vi "PlainTextToVariant.vi"(7 "use system decimal point (T)":bool=TRUE, 11 "String-formatted Value":string) -> (2 "Value Class":T1, 3 "Variant-formatted Value":variant)   [LabVIEW 2013, in "OpenSerializer.lvlib" / "Serializer.PlainText.lvclass"]
uses:
  Serializer.PlainText.lvclass
  Character Class -- Enum.ctl
  <vilib>/LabVIEW Open Source Project/Data Manipulation/Variant/Variant_EmptyCluster.vi
  <vilib>/Utility/GetType.llb/TD_Create Cluster.vi
  <vilib>/LabVIEW Open Source Project/Data Manipulation/Variant/OpenVariant.lvlib
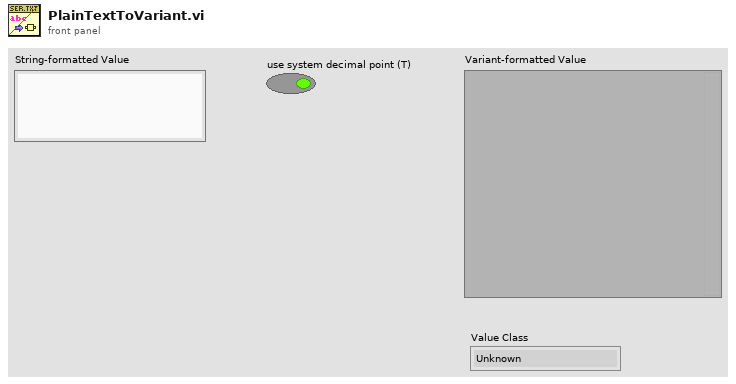
[diagram p1: front panel]
types:
  T1 = typedef "OpenSerializer.lvlib/Serializer.PlainText.lvclass/Character Class -- Enum.ctl" = enum16{"Unknown", "Sign", "Zero", "Integer", "Float", "Complex", "Scientific", "Engineering", "Hexadecimal", "Binary", "Decimal", "Octal", "Unit", "Invalid", "Timestamp", "Boolean", "String", "Path", "null", "cluster", "array"}
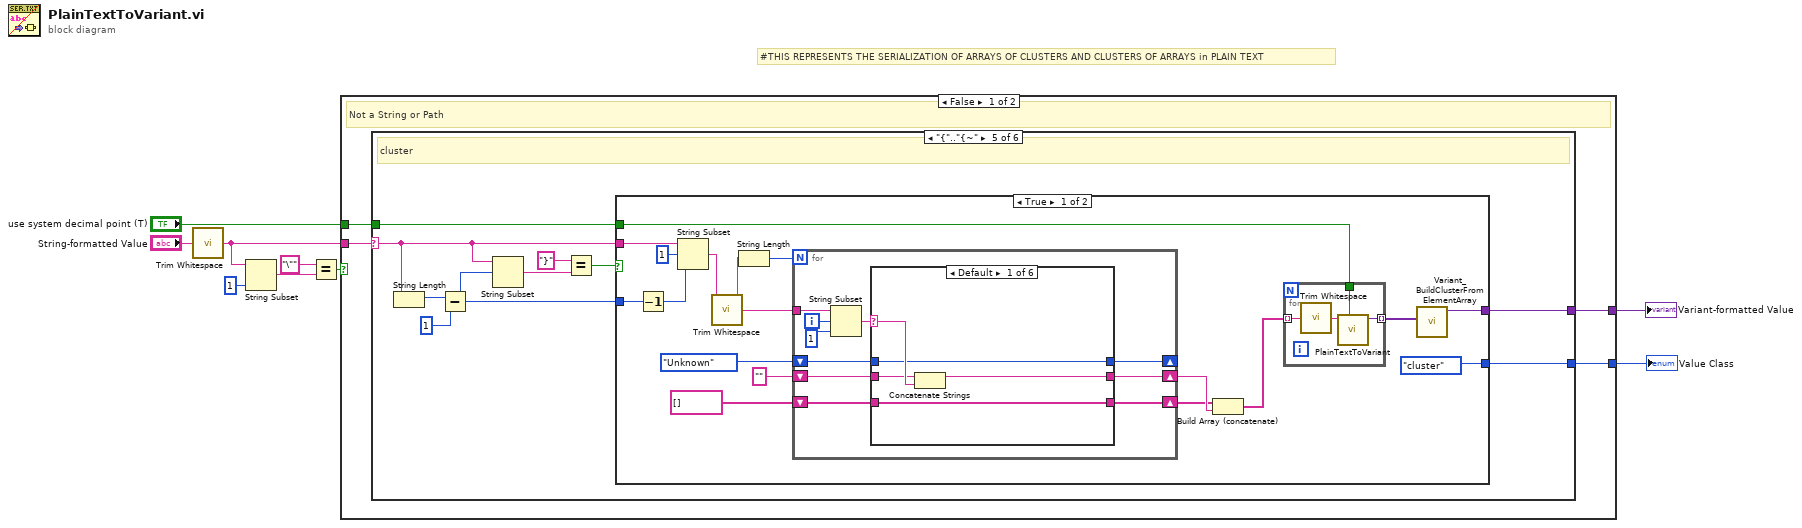
[diagram p0: block diagram]
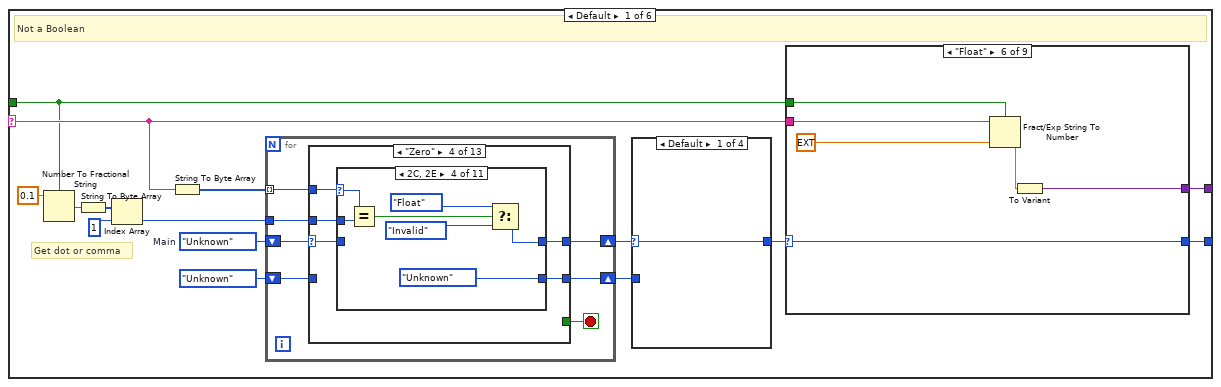
[diagram p2: hidden frame]
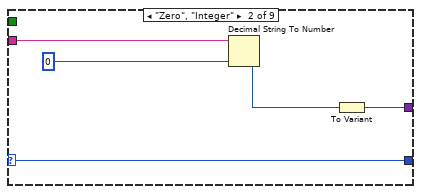
[diagram p4: hidden frame]
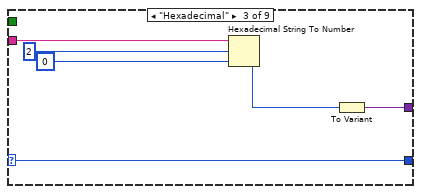
[diagram p5: hidden frame]
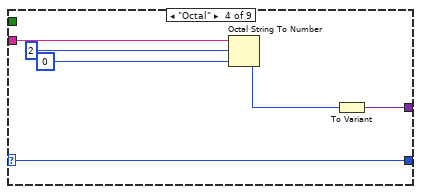
[diagram p6: hidden frame]
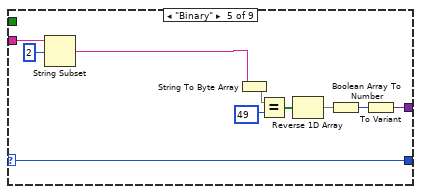
[diagram p7: hidden frame]
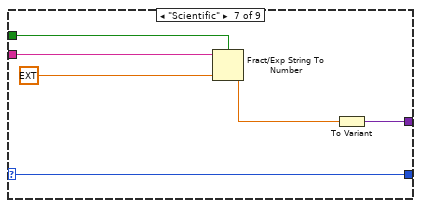
[diagram p8: hidden frame]
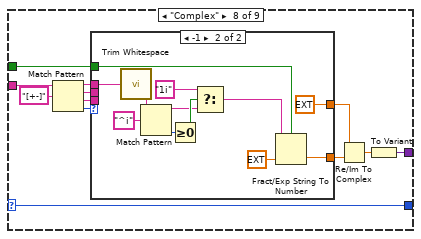
[diagram p9: hidden frame]
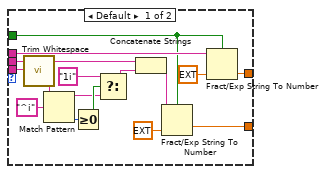
[diagram p10: hidden frame]
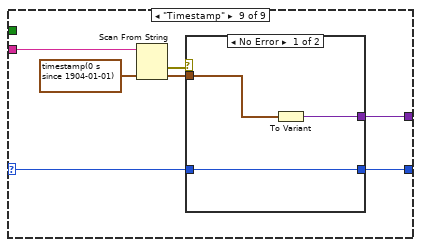
[diagram p11: hidden frame]
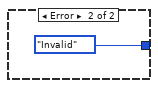
[diagram p12: hidden frame]
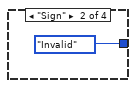
[diagram p13: hidden frame]
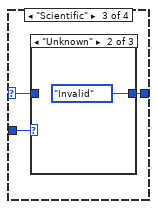
[diagram p14: hidden frame]
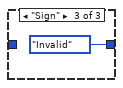
[diagram p16: hidden frame]
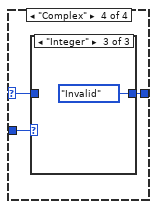
[diagram p17: hidden frame]
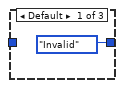
[diagram p18: hidden frame]
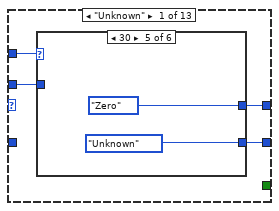
[diagram p20: hidden frame]
diagram:
  # "#THIS REPRESENTS THE SERIALIZATION OF ARRAYS OF CLUSTERS AND CLUSTERS OF ARRAYS in PLAIN TEXT"
  n1 = call <vilib>:"Trim Whitespace.vi"("string"="String-formatted Value") -> ("trimmed string"=w8:string)  [unwired: 1 in]
  n2 = String Subset(string=w8, length (rest)=1 ("length (rest)")) -> (substring=w6:string)  [unwired: 1 in]
  n3 = Equal?(x="\"", y=w6) -> (x = y?=w4:bool)
  n4 = case shown="False" w4 {
    tunnel: w8 -> [w13 w620]
    tunnel: [w12 w628] -> w9
    tunnel: [w11 w621] -> w3
    tunnel: "use system decimal point (T)" -> [w10 _]
    frame False {
      # "Not a String or Path"
      n5 = case shown="\"{\"..\"{~\"" w13 {
        selector: w13 -> [w23 _ _ _ w387 w507]
        tunnel: [w22 w374 w377 w381 w391 w511] -> w12
        tunnel: [w21 Character_Class_--_Enum."Boolean" Character_Class_--_Enum."Boolean" Character_Class_--_Enum."null" w390 w510] -> w11
        tunnel: w10 -> [w18 _ _ _ w382 w502]
        frame Default {
          w27 = Character_Class_--_Enum."Unknown"  # Main
          # "Get dot or comma"
          # "Not a Boolean"
          n6 = Number To Fractional String(use system decimal point (T)=w18, number=0.1) -> (F-format string=w16:string)  [unwired: 2 in]
          n7 = String To Byte Array(string=w16) -> (unsigned byte array=w17:u8[])
          n8 = Index Array(array=w17, index=1 ("length (rest)")) -> (element=w14:u8)
          n9 = String To Byte Array(string=w23) -> (unsigned byte array=w28:u8[])
          n10 = for {
            tunnel: w28 -> [w139] mode=indexing
            shift-right: [w138] -> w26
            shift-left: w27 -> [w140]
            shift-right: [w136] -> w25
            shift-left: Character_Class_--_Enum."Unknown" -> [w137]
            tunnel: w14 -> [w134]
            stop <- w135 stop-if-true
            n11 = case shown="\"Zero\"" w140 {
              selector: w140 -> [_ w163 w167 w186 w217 w240 w246 w252 w258 w264 w267 w283 w324]
              tunnel: w139 -> [w144 _ w169 w188 w219 w242 w248 w254 w260 _ w269 w285 w326]
              tunnel: [w143 w163 w168 w187 w218 w241 w247 w253 w259 w264 w268 w284 w325] -> w138
              tunnel: w137 -> [_ w162 w164 _ _ _ _ _ _ _ _ w282 w323]
              tunnel: [w142 w162 w165 w185 w216 Character_Class_--_Enum."Unknown" Character_Class_--_Enum."Unknown" Character_Class_--_Enum."Unknown" Character_Class_--_Enum."Unknown" Character_Class_--_Enum."Unknown" w266 w281 w322] -> w136
              tunnel: [_ TRUE _ _ _ _ _ _ _ TRUE _ _ _] -> w135
              tunnel: w134 -> [w141 _ w166 w184 w215 _ _ _ _ _ _ _ w321]
              frame "Unknown" {
                n12 = case shown="30" w144 {
                  selector: w144 -> [_ _ _ w155 _ _]
                  tunnel: [Character_Class_--_Enum."Invalid" Character_Class_--_Enum."Sign" Character_Class_--_Enum."Integer" w151 Character_Class_--_Enum."Zero" w160] -> w143
                  tunnel: [Character_Class_--_Enum."Unknown" Character_Class_--_Enum."Unknown" Character_Class_--_Enum."Unknown" Character_Class_--_Enum."Unknown" Character_Class_--_Enum."Unknown" w160] -> w142
                  tunnel: w141 -> [_ _ _ w156 _ _]
                  frame Default {
                  }
                  frame 43, 45 {
                  }
                  frame 49..57 {
                  }
                  frame 44, 46 {
                    n13 = Equal?(x=w155, y=w156) -> (x = y?=w154:bool)
                    n14 = Select(t=Character_Class_--_Enum."Float", s=w154, f=Character_Class_--_Enum."Invalid") -> (s? t:f=w151:T1)
                  }
                  frame 48 {
                  }
                  frame 105 {
                    w160 = Character_Class_--_Enum."Complex"
                  }
                }
              }
              frame "Invalid", Default {
              }
              frame "Sign" {
                n15 = case shown="69" w169 {
                  selector: w169 -> [_ _ _ _ w180]
                  tunnel: [Character_Class_--_Enum."Invalid" w173 Character_Class_--_Enum."Integer" w176 w178] -> w168
                  tunnel: w167 -> [_ w173 _ _ _]
                  tunnel: w166 -> [_ _ _ _ w179]
                  tunnel: [Character_Class_--_Enum."Unknown" w172 Character_Class_--_Enum."Unknown" w176 Character_Class_--_Enum."Unknown"] -> w165
                  tunnel: w164 -> [_ w172 _ _ _]
                  frame Default {
                  }
                  frame 32 {
                    # "space (ignore)"
                  }
                  frame 48..57 {
                  }
                  frame 105 {
                    w176 = Character_Class_--_Enum."Complex"
                  }
                  frame 44, 46 {
                    n16 = Equal?(x=w180, y=w179) -> (x = y?=w183:bool)
                    n17 = Select(t=Character_Class_--_Enum."Float", s=w183, f=Character_Class_--_Enum."Invalid") -> (s? t:f=w178:T1)
                  }
                }
              }
              frame "Zero" {
                n18 = case shown="2C, 2E" w188 {
                  selector: w188 -> [_ _ _ w196 _ _ _ _ _ _ _]
                  tunnel: [Character_Class_--_Enum."Invalid" Character_Class_--_Enum."Integer" w194 w195 Character_Class_--_Enum."Hexadecimal" Character_Class_--_Enum."Binary" Character_Class_--_Enum."Octal" Character_Class_--_Enum."Decimal" w211 w212 Character_Class_--_Enum."Complex"] -> w187
                  tunnel: w186 -> [_ _ w194 _ _ _ _ _ w211 _ _]
                  tunnel: [Character_Class_--_Enum."Unknown" Character_Class_--_Enum."Unknown" Character_Class_--_Enum."Unknown" Character_Class_--_Enum."Unknown" Character_Class_--_Enum."Unknown" Character_Class_--_Enum."Unknown" Character_Class_--_Enum."Unknown" Character_Class_--_Enum."Unknown" Character_Class_--_Enum."Unknown" w212 Character_Class_--_Enum."Unknown"] -> w185
                  tunnel: w184 -> [_ _ _ w197 _ _ _ _ _ _ _]
                  frame Default {
                  }
                  frame 49..57 {
                  }
                  frame 48 {
                  }
                  frame 44, 46 {
                    n19 = Equal?(x=w196, y=w197) -> (x = y?=w200:bool)
                    n20 = Select(t=Character_Class_--_Enum."Float", s=w200, f=Character_Class_--_Enum."Invalid") -> (s? t:f=w195:T1)
                  }
                  frame 120 {
                  }
                  frame 98 {
                  }
                  frame 111 {
                  }
                  frame 100 {
                  }
                  frame 32 {
                  }
                  frame 105 {
                    w212 = Character_Class_--_Enum."Complex"
                  }
                  frame 43, 45 {
                  }
                }
              }
              frame "Integer" {
                n21 = case shown="3A" w219 {
                  selector: w219 -> [_ _ _ _ _ w230 _ _]
                  tunnel: [Character_Class_--_Enum."Invalid" w222 w223 w225 w227 w228 Character_Class_--_Enum."Complex" Character_Class_--_Enum."Scientific"] -> w218
                  tunnel: w217 -> [_ _ _ w225 w227 _ _ _]
                  tunnel: [Character_Class_--_Enum."Unknown" w222 w223 Character_Class_--_Enum."Unknown" Character_Class_--_Enum."Unknown" Character_Class_--_Enum."Unknown" Character_Class_--_Enum."Unknown" Character_Class_--_Enum."Unknown"] -> w216
                  tunnel: w215 -> [_ _ _ _ _ w229 _ _]
                  frame Default {
                  }
                  frame 105 {
                    w222 = Character_Class_--_Enum."Complex"
                  }
                  frame 58 {
                    w223 = Character_Class_--_Enum."Timestamp"
                  }
                  frame 32 {
                  }
                  frame 48..57 {
                  }
                  frame 44, 46 {
                    n22 = Equal?(x=w230, y=w229) -> (x = y?=w233:bool)
                    n23 = Select(t=Character_Class_--_Enum."Float", s=w233, f=Character_Class_--_Enum."Invalid") -> (s? t:f=w228:T1)
                  }
                  frame 43, 45 {
                  }
                  frame 69, 101 {
                  }
                }
              }
              frame "Hexadecimal" {
                n24 = case shown="30..39, 41..46" w242 {
                  tunnel: [Character_Class_--_Enum."Invalid" w244] -> w241
                  tunnel: w240 -> [_ w244]
                  frame Default {
                  }
                  frame 48..57, 65..70 {
                  }
                }
              }
              frame "Decimal" {
                n25 = case shown="30..39" w248 {
                  tunnel: [Character_Class_--_Enum."Invalid" w250] -> w247
                  tunnel: w246 -> [_ w250]
                  frame Default {
                  }
                  frame 48..57 {
                  }
                }
              }
              frame "Octal" {
                n26 = case shown="30..37" w254 {
                  tunnel: [Character_Class_--_Enum."Invalid" w256] -> w253
                  tunnel: w252 -> [_ w256]
                  frame Default {
                  }
                  frame 48..55 {
                  }
                }
              }
              frame "Binary" {
                n27 = case shown="30, 31" w260 {
                  tunnel: [Character_Class_--_Enum."Invalid" w262] -> w259
                  tunnel: w258 -> [_ w262]
                  frame Default {
                  }
                  frame 48, 49 {
                  }
                }
              }
              frame "Timestamp" {
              }
              frame "Float" {
                n28 = case shown="2B, 2D" w269 {
                  tunnel: [Character_Class_--_Enum."Invalid" w273 Character_Class_--_Enum."Scientific" w277 Character_Class_--_Enum."Complex" w280] -> w268
                  tunnel: w267 -> [_ w273 _ w277 _ _]
                  tunnel: [Character_Class_--_Enum."Unknown" Character_Class_--_Enum."Unknown" Character_Class_--_Enum."Unknown" Character_Class_--_Enum."Unknown" Character_Class_--_Enum."Unknown" w280] -> w266
                  frame Default {
                  }
                  frame 48..57 {
                  }
                  frame 69, 101 {
                  }
                  frame 32 {
                  }
                  frame 43, 45 {
                  }
                  frame 105 {
                    w280 = Character_Class_--_Enum."Complex"
                  }
                }
              }
              frame "Scientific" {
                n29 = case shown="2B, 2D" w285 {
                  tunnel: [Character_Class_--_Enum."Invalid" w289 w301 w314] -> w284
                  tunnel: w283 -> [_ w288 w303 w316]
                  tunnel: w282 -> [w286 w290 w302 w315]
                  tunnel: [w286 w291 w304 w317] -> w281
                  frame Default {
                  }
                  frame 49..57 {
                    n30 = case shown="\"Unknown\"" w290 {
                      selector: w290 -> [_ _ _ w297 _]
                      tunnel: [w292 Character_Class_--_Enum."Integer" Character_Class_--_Enum."Integer" w297 Character_Class_--_Enum."Integer"] -> w291
                      tunnel: [w292 w293 w296 w298 w300] -> w289
                      tunnel: w288 -> [_ w293 w296 w298 w300]
                      frame Default {
                        w292 = Character_Class_--_Enum."Invalid"
                      }
                      frame "Sign" {
                      }
                      frame "Zero" {
                      }
                      frame "Integer" {
                      }
                      frame "Unknown" {
                      }
                    }
                  }
                  frame 48 {
                    n31 = case shown="\"Sign\"" w302 {
                      tunnel: [w305 Character_Class_--_Enum."Zero" Character_Class_--_Enum."Zero" Character_Class_--_Enum."Zero" Character_Class_--_Enum."Integer"] -> w304
                      tunnel: w303 -> [_ w306 w308 w310 w312]
                      tunnel: [w305 w306 w308 w310 w312] -> w301
                      frame Default {
                        w305 = Character_Class_--_Enum."Invalid"
                      }
                      frame "Unknown" {
                      }
                      frame "Sign" {
                      }
                      frame "Zero" {
                      }
                      frame "Integer" {
                      }
                    }
                  }
                  frame 43, 45 {
                    n32 = case shown="\"Unknown\"" w315 {
                      tunnel: [w318 Character_Class_--_Enum."Sign"] -> w317
                      tunnel: w316 -> [_ w319]
                      tunnel: [w318 w319] -> w314
                      frame Default {
                        w318 = Character_Class_--_Enum."Invalid"
                      }
                      frame "Unknown" {
                      }
                    }
                  }
                }
              }
              frame "Complex" {
                n33 = case shown="2C, 2E" w326 {
                  selector: w326 -> [_ _ _ w342 _]
                  tunnel: [w327 w329 w332 w345 w364] -> w325
                  tunnel: w324 -> [_ w329 w330 w343 w362]
                  tunnel: w323 -> [_ w328 w333 w346 w365]
                  tunnel: [w327 w328 w331 w344 w363] -> w322
                  tunnel: w321 -> [_ _ _ w341 _]
                  frame Default {
                    w327 = Character_Class_--_Enum."Invalid"
                  }
                  frame 32 {
                  }
                  frame 48..57 {
                    n34 = case shown="Default" w333 {
                      selector: w333 -> [_ _ w337 w339]
                      tunnel: [w334 w336 w338 w340] -> w332
                      tunnel: [w334 Character_Class_--_Enum."Integer" w337 w339] -> w331
                      tunnel: w330 -> [_ w336 w338 w340]
                      frame Default {
                        w334 = Character_Class_--_Enum."Invalid"
                      }
                      frame "Unknown" {
                      }
                      frame "Integer" {
                      }
                      frame "Float" {
                      }
                    }
                  }
                  frame 44, 46 {
                    n35 = case shown="\"Unknown\"" w346 {
                      tunnel: [w347 w354 w361] -> w345
                      tunnel: [w347 w348 w357] -> w344
                      tunnel: w343 -> [_ w354 w361]
                      tunnel: w342 -> [_ w350 w356]
                      tunnel: w341 -> [_ w349 w355]
                      frame Default {
                        w347 = Character_Class_--_Enum."Invalid"
                      }
                      frame "Unknown" {
                        n36 = Equal?(x=w350, y=w349) -> (x = y?=w353:bool)
                        n37 = Select(t=Character_Class_--_Enum."Float", s=w353, f=Character_Class_--_Enum."Invalid") -> (s? t:f=w348:T1)
                      }
                      frame "Integer" {
                        n38 = Equal?(x=w356, y=w355) -> (x = y?=w360:bool)
                        n39 = Select(t=Character_Class_--_Enum."Float", s=w360, f=Character_Class_--_Enum."Invalid") -> (s? t:f=w357:T1)
                      }
                    }
                  }
                  frame 105 {
                    n40 = case shown="\"Float\"" w365 {
                      tunnel: [w366 w368 w370 w372] -> w364
                      tunnel: [w366 Character_Class_--_Enum."Complex" Character_Class_--_Enum."Complex" Character_Class_--_Enum."Complex"] -> w363
                      tunnel: w362 -> [_ w368 w370 w372]
                      frame Default {
                        w366 = Character_Class_--_Enum."Invalid"
                      }
                      frame "Unknown" {
                      }
                      frame "Integer" {
                      }
                      frame "Float" {
                      }
                    }
                  }
                }
              }
            }
          }
          n41 = case shown="Default" w26 {
            selector: w26 -> [w120 _ w122 w128]
            tunnel: w25 -> [_ _ w124 w130]
            tunnel: [w120 Character_Class_--_Enum."Invalid" w123 w129] -> w24
            frame Default {
            }
            frame "Sign" {
            }
            frame "Scientific" {
              n42 = case shown="\"Unknown\"" w124 {
                tunnel: [w125 Character_Class_--_Enum."Invalid" Character_Class_--_Enum."Invalid"] -> w123
                tunnel: w122 -> [w125 _ _]
                frame Default {
                }
                frame "Unknown" {
                }
                frame "Sign" {
                }
              }
            }
            frame "Complex" {
              n43 = case shown="\"Integer\"" w130 {
                tunnel: [Character_Class_--_Enum."Invalid" w132 Character_Class_--_Enum."Invalid" ("Main")] -> w129
                tunnel: w128 -> [_ w132 _]
                frame Default {
                }
                frame "Complex" {
                }
                frame "Integer" {
                }
              }
            }
          }
          n44 = case shown="\"Float\"" w24 {
            selector: w24 -> [w29 w30 w35 w41 w47 w58 w64 w79 w109]
            tunnel: w23 -> [_ w34 w40 w46 w55 w62 w68 w75 w115]
            tunnel: [_ w31 w37 w43 w56 w59 w65 w80 w112] -> w22
            tunnel: [w29 w30 w35 w41 w47 w58 w64 w79 w110] -> w21
            tunnel: w18 -> [_ _ _ _ _ w57 w63 w70 _]
            frame Default {
            }
            frame "Zero", "Integer" {
              n45 = Decimal String To Number(string=w34, default (0L)=i64 0 ("default (0 I32)")) -> (number=w32:i64)  [unwired: 1 in, 1 out]
              n46 = To Variant(anything=w32) -> (Variant=w31:variant)
            }
            frame "Hexadecimal" {
              n47 = Hexadecimal String To Number(string=w40, offset=2, default (0uL)=i64 0 ("default (0 I32)")) -> (number=w38:i64)  [unwired: 1 out]
              n48 = To Variant(anything=w38) -> (Variant=w37:variant)
            }
            frame "Octal" {
              n49 = Octal String To Number(2:i64 0 ("default (0 I32)"), 3:2 ("offset"), 4:w46) -> (0:w44:i64)  [unwired: 1 out]
              n50 = To Variant(anything=w44) -> (Variant=w43:variant)
            }
            frame "Binary" {
              n51 = String Subset(string=w55, offset (0)=2) -> (substring=w53:string)  [unwired: 1 in]
              n52 = String To Byte Array(string=w53) -> (unsigned byte array=w51:u8[])
              n53 = Equal?(x=w51, y=u8 49 ("offset (0)")) -> (x = y?=w50:bool[])
              n54 = Reverse 1D Array(array=w50) -> (reversed array=w48:bool[])
              n55 = Boolean Array To Number(Boolean array=w48) -> (number=w52:u32)
              n56 = To Variant(anything=w52) -> (Variant=w56:variant)
            }
            frame "Float" {
              n57 = Fract/Exp String To Number(use system decimal point (T)=w57, string=w62, default (0 dbl)=ext 0.0 ("default (0 I32)")) -> (number=w60:ext)  [unwired: 1 in, 1 out]
              n58 = To Variant(anything=w60) -> (Variant=w59:variant)
            }
            frame "Scientific" {
              n59 = Fract/Exp String To Number(use system decimal point (T)=w63, string=w68, default (0 dbl)=ext 0.0 ("default (0 I32)")) -> (number=w66:ext)  [unwired: 1 in, 1 out]
              n60 = To Variant(anything=w66) -> (Variant=w65:variant)
            }
            frame "Complex" {
              n61 = Match Pattern(string=w75, regular expression="[+-]") -> (before substring=w72:string, match substring=w69:string, after substring=w71:string, offset past match=w76:i32)  [unwired: 1 in]
              n62 = case shown="-1" w76 {
                tunnel: [w93 ext 0.0 ("default (0 DBL)")] -> w73
                tunnel: [w95 w106] -> w74
                tunnel: w72 -> [w92 w98]
                tunnel: w71 -> [w82 _]
                tunnel: w70 -> [w91 w105]
                tunnel: w69 -> [w85 _]
                frame Default {
                  n63 = call <vilib>:"Trim Whitespace.vi"("string"=w82) -> ("trimmed string"=w83:string)  [unwired: 1 in]
                  n64 = Match Pattern(string=w83, regular expression="^i") -> (before substring=w88:string, offset past match=w90:i32)  [unwired: 1 in, 2 out]
                  n65 = Greater Or Equal To 0?(x=w90) -> (x >= 0?=w89:bool)
                  n66 = Select(t="1i", s=w89, f=w88) -> (s? t:f=w86:string)
                  n67 = Concatenate Strings(w85, w86) -> (w84:string)
                  n68 = Fract/Exp String To Number(use system decimal point (T)=w91, string=w84, default (0 dbl)=ext 0.0 ("default (0 DBL)")) -> (number=w95:ext)  [unwired: 1 in, 1 out]
                  n69 = Fract/Exp String To Number(use system decimal point (T)=w91, string=w92, default (0 dbl)=ext 0.0 ("default (0 DBL)")) -> (number=w93:ext)  [unwired: 1 in, 1 out]
                }
                frame -1 {
                  n70 = call <vilib>:"Trim Whitespace.vi"("string"=w98) -> ("trimmed string"=w100:string)  [unwired: 1 in]
                  n71 = Match Pattern(string=w100, regular expression="^i") -> (before substring=w102:string, offset past match=w104:i32)  [unwired: 1 in, 2 out]
                  n72 = Greater Or Equal To 0?(x=w104) -> (x >= 0?=w103:bool)
                  n73 = Select(t="1i", s=w103, f=w102) -> (s? t:f=w97:string)
                  n74 = Fract/Exp String To Number(use system decimal point (T)=w105, string=w97, default (0 dbl)=ext 0.0 ("default (0 DBL)")) -> (number=w106:ext)  [unwired: 1 in, 1 out]
                }
              }
              n75 = Re/Im To Complex(1:w74, 2:w73) -> (0:w78:cxt)
              n76 = To Variant(anything=w78) -> (Variant=w80:variant)
            }
            frame "Timestamp" {
              n77 = Scan From String(input string=w115, default 1=timestamp(0 s since 1904-01-01)) -> (error out=w111:errorcluster, output 1=w113:timestamp)  [unwired: 3 in, 2 out]
              n78 = case shown="No Error" w111 {
                tunnel: w113 -> [w118 _]
                tunnel: [w117 _] -> w112
                tunnel: [w116 Character_Class_--_Enum."Invalid"] -> w110
                tunnel: w109 -> [w116 _]
                frame No Error {
                  n79 = To Variant(anything=w118) -> (Variant=w117:variant)
                }
                frame Error {
                }
              }
            }
          }
        }
        frame "true" {
          # "BOOLEAN (TRUE)"
          n80 = To Variant(anything=TRUE) -> (Variant=w374:variant)
        }
        frame "false" {
          # "BOOLEAN (FALSE)"
          n81 = To Variant(anything=FALSE) -> (Variant=w377:variant)
        }
        frame "null" {
          # "null"
          n82 = To Variant(anything=variant ("variant")) -> (Variant=w381:variant)
        }
        frame "{".."{~" {
          # "cluster"
          n83 = String Length(string=w387) -> (length=w389:i32)
          n84 = Subtract(x=w389, y=1) -> (x-y=w383:i32)
          n85 = String Subset(string=w387, offset (0)=w383) -> (substring=w385:string)  [unwired: 1 in]
          n86 = Equal?(x="}", y=w385) -> (x = y?=w384:bool)
          n87 = case shown="True" w384 {
            tunnel: [w400 w501] -> w391
            tunnel: [Character_Class_--_Enum."cluster" Character_Class_--_Enum."Invalid"] -> w390
            tunnel: w387 -> [w407 _]
            tunnel: w383 -> [w405 _]
            tunnel: w382 -> [w402 _]
            frame True {
              n88 = Decrement(x=w405) -> (x-1=w404:i32)
              n89 = String Subset(string=w407, offset (0)=1, length (rest)=w404) -> (substring=w403:string)
              n90 = call <vilib>:"Trim Whitespace.vi"("string"=w403) -> ("trimmed string"=w397:string)  [unwired: 1 in]
              n91 = String Length(string=w397) -> (length=w398:i32)
              n92 = for {
                N: w398 -> [_]
                shift-right: [w412] -> w394
                shift-left: string[] [] -> [w413]
                tunnel: w397 -> [w418]
                shift-right: [w411] -> w395
                shift-left: "" -> [w414]
                shift-right: [w409] -> _
                shift-left: Character_Class_--_Enum."Unknown" -> [w410]
                i -> [w417]
                n93 = String Subset(string=w418, offset (0)=w417, length (rest)=1 ("offset (0)")) -> (substring=w415:string)
                n94 = case shown="Default" w415 {
                  selector: w415 -> [w422 w425 w443 w455 w469 w483]
                  tunnel: w414 -> [w421 w430 w444 w456 w470 w484]
                  tunnel: w413 -> [w423 w429 w446 w458 w472 w486]
                  tunnel: [w423 w428 w446 w458 w472 w486] -> w412
                  tunnel: [w420 w427 w442 w454 w468 w482] -> w411
                  tunnel: w410 -> [w419 w426 w445 w457 w471 w485]
                  tunnel: [w419 w424 w441 w453 w467 w481] -> w409
                  frame Default {
                    n95 = Concatenate Strings(w421, w422) -> (w420:string)
                  }
                  frame "," {
                    n96 = case shown="\"Unknown\", Default" w426 {
                      selector: w426 -> [w431 w436]
                      tunnel: w430 -> [w435 w439]
                      tunnel: w429 -> [w434 w440]
                      tunnel: [w433 w440] -> w428
                      tunnel: ["" w437] -> w427
                      tunnel: w425 -> [_ w438]
                      tunnel: [w431 w436] -> w424
                      frame "Unknown", Default {
                        n97 = Build Array (concatenate)(w434, w435) -> (w433:string[])
                      }
                      frame "cluster", "array" {
                        n98 = Concatenate Strings(w439, w438) -> (w437:string)
                      }
                    }
                  }
                  frame "{" {
                    n99 = case shown="Default" w445 {
                      selector: w445 -> [_ w449]
                      tunnel: w444 -> [_ w452]
                      tunnel: w443 -> [w447 w451]
                      tunnel: [w447 w450] -> w442
                      tunnel: [Character_Class_--_Enum."cluster" w449] -> w441
                      frame Default {
                      }
                      frame "cluster" {
                        n100 = Concatenate Strings(w452, w451) -> (w450:string)
                      }
                    }
                  }
                  frame "}" {
                    n101 = case shown="\"cluster\"" w457 {
                      selector: w457 -> [w459 _]
                      tunnel: w456 -> [w462 w464]
                      tunnel: w455 -> [w461 w465]
                      tunnel: [w460 w463] -> w454
                      tunnel: [w459 Character_Class_--_Enum."Unknown"] -> w453
                      frame Default {
                        n102 = Concatenate Strings(w462, w461) -> (w460:string)
                      }
                      frame "cluster" {
                        n103 = Concatenate Strings(w464, w465) -> (w463:string)
                      }
                    }
                  }
                  frame "[" {
                    n104 = case shown="Default" w471 {
                      tunnel: w470 -> [w476 w478]
                      tunnel: w469 -> [w475 w479]
                      tunnel: [w474 w477] -> w468
                      tunnel: [Character_Class_--_Enum."array" Character_Class_--_Enum."array"] -> w467
                      frame Default {
                        n105 = Concatenate Strings(w476, w475) -> (w474:string)
                      }
                      frame "cluster" {
                        n106 = Concatenate Strings(w478, w479) -> (w477:string)
                      }
                    }
                  }
                  frame "]" {
                    n107 = case shown="\"array\"" w485 {
                      selector: w485 -> [w487 _]
                      tunnel: w484 -> [w490 w492]
                      tunnel: w483 -> [w489 w493]
                      tunnel: [w488 w491] -> w482
                      tunnel: [w487 Character_Class_--_Enum."Unknown"] -> w481
                      frame Default {
                        n108 = Concatenate Strings(w490, w489) -> (w488:string)
                      }
                      frame "array" {
                        n109 = Concatenate Strings(w492, w493) -> (w491:string)
                      }
                    }
                  }
                }
              }
              n110 = Build Array (concatenate)(w394, w395) -> (w393:string[])
              n111 = for {
                tunnel: w402 -> [w498]
                tunnel: w393 -> [w497] mode=indexing
                tunnel: [w495] -> w401 mode=indexing
                n112 = call <vilib>:"Trim Whitespace.vi"("string"=w497) -> ("trimmed string"=w496:string)  [unwired: 1 in]
                n113 = call "PlainTextToVariant.vi"("use system decimal point (T)"=w498, "String-formatted Value"=w496) -> ("Variant-formatted Value"=w495:variant)  [unwired: 8 in, 1 out]
              }
              n114 = call <vilib>:"Variant_BuildClusterFromElementArray.vi"("Elements"=w401) -> ("Cluster"=w400:variant)  [unwired: 10 in]
            }
            frame False {
              n115 = To Variant(anything=variant ("variant")) -> (Variant=w501:variant)
            }
          }
        }
        frame "[".."[~" {
          # "array"
          n116 = String Length(string=w507) -> (length=w509:i32)
          n117 = Subtract(x=w509, y=1) -> (x-y=w503:i32)
          n118 = String Subset(string=w507, offset (0)=w503) -> (substring=w505:string)  [unwired: 1 in]
          n119 = Equal?(x="]", y=w505) -> (x = y?=w504:bool)
          n120 = case shown="True" w504 {
            tunnel: [w515 w619] -> w511
            tunnel: [Character_Class_--_Enum."array" Character_Class_--_Enum."Invalid"] -> w510
            tunnel: w507 -> [w513 _]
            tunnel: w503 -> [w526 _]
            tunnel: w502 -> [w524 _]
            frame True {
              # "#THIS IS UPDATED AS WELL\nto support undefined array input"
              n121 = Decrement(x=w526) -> (x-1=w525:i32)
              n122 = String Subset(string=w513, offset (0)=1, length (rest)=w525) -> (substring=w512:string)
              n123 = call <vilib>:"Trim Whitespace.vi"("string"=w512) -> ("trimmed string"=w521:string)  [unwired: 1 in]
              n124 = String Length(string=w521) -> (length=w522:i32)
              n125 = for {
                N: w522 -> [_]
                shift-right: [w532] -> w518
                shift-left: string[] [] -> [w533]
                tunnel: w521 -> [w538]
                shift-right: [w531] -> w519
                shift-left: "" -> [w534]
                shift-right: [w529] -> _
                shift-left: Character_Class_--_Enum."Unknown" -> [w530]
                i -> [w537]
                n126 = String Subset(string=w538, offset (0)=w537, length (rest)=1 ("offset (0)")) -> (substring=w535:string)
                n127 = case shown="\"]\"" w535 {
                  selector: w535 -> [w542 w545 w563 w575 w587 w601]
                  tunnel: w534 -> [w541 w550 w564 w576 w588 w602]
                  tunnel: w533 -> [w543 w549 w566 w578 w590 w604]
                  tunnel: [w543 w548 w566 w578 w590 w604] -> w532
                  tunnel: [w540 w547 w562 w574 w586 w600] -> w531
                  tunnel: w530 -> [w539 w546 w565 w577 w589 w603]
                  tunnel: [w539 w544 w561 w573 w585 w599] -> w529
                  frame Default {
                    n128 = Concatenate Strings(w541, w542) -> (w540:string)
                  }
                  frame "," {
                    n129 = case shown="\"cluster\"" w546 {
                      selector: w546 -> [w551 w556]
                      tunnel: w550 -> [w555 w559]
                      tunnel: w549 -> [w554 w560]
                      tunnel: [w553 w560] -> w548
                      tunnel: ["" w557] -> w547
                      tunnel: w545 -> [_ w558]
                      tunnel: [w551 w556] -> w544
                      frame "Unknown", Default {
                        n130 = Build Array (concatenate)(w554, w555) -> (w553:string[])
                      }
                      frame "cluster" {
                        n131 = Concatenate Strings(w559, w558) -> (w557:string)
                      }
                    }
                  }
                  frame "[" {
                    n132 = case shown="\"array\"" w565 {
                      selector: w565 -> [_ w569]
                      tunnel: w564 -> [_ w572]
                      tunnel: w563 -> [w567 w571]
                      tunnel: [w567 w570] -> w562
                      tunnel: [Character_Class_--_Enum."array" w569] -> w561
                      frame Default {
                      }
                      frame "array" {
                        n133 = Concatenate Strings(w572, w571) -> (w570:string)
                      }
                    }
                  }
                  frame "{" {
                    n134 = case shown="Default" w577 {
                      selector: w577 -> [_ w581]
                      tunnel: w576 -> [_ w584]
                      tunnel: w575 -> [w579 w583]
                      tunnel: [w579 w582] -> w574
                      tunnel: [Character_Class_--_Enum."cluster" w581] -> w573
                      frame Default {
                      }
                      frame "cluster" {
                        n135 = Concatenate Strings(w584, w583) -> (w582:string)
                      }
                    }
                  }
                  frame "]" {
                    n136 = case shown="\"array\"" w589 {
                      selector: w589 -> [w591 _]
                      tunnel: w588 -> [w594 w596]
                      tunnel: w587 -> [w593 w597]
                      tunnel: [w592 w595] -> w586
                      tunnel: [w591 Character_Class_--_Enum."Unknown"] -> w585
                      frame Default {
                        n137 = Concatenate Strings(w594, w593) -> (w592:string)
                      }
                      frame "array" {
                        n138 = Concatenate Strings(w596, w597) -> (w595:string)
                      }
                    }
                  }
                  frame "}" {
                    n139 = case shown="\"cluster\"" w603 {
                      selector: w603 -> [w605 _]
                      tunnel: w602 -> [w608 w610]
                      tunnel: w601 -> [w607 w611]
                      tunnel: [w606 w609] -> w600
                      tunnel: [w605 Character_Class_--_Enum."Unknown"] -> w599
                      frame Default {
                        n140 = Concatenate Strings(w608, w607) -> (w606:string)
                      }
                      frame "cluster" {
                        n141 = Concatenate Strings(w610, w611) -> (w609:string)
                      }
                    }
                  }
                }
              }
              n142 = Build Array (concatenate)(w518, w519) -> (w517:string[])
              n143 = for {
                tunnel: w524 -> [w616]
                tunnel: w517 -> [w615] mode=indexing
                tunnel: [w613] -> w514 mode=indexing
                n144 = call <vilib>:"Trim Whitespace.vi"("string"=w615) -> ("trimmed string"=w614:string)  [unwired: 1 in]
                n145 = call "PlainTextToVariant.vi"("use system decimal point (T)"=w616, "String-formatted Value"=w614) -> ("Variant-formatted Value"=w613:variant)  [unwired: 8 in, 1 out]
              }
              n146 = call <vilib>:"Variant_BuildArrayFromElementArray.vi"("Elements"=w514) -> ("Output Array"=w515:variant)  [unwired: 9 in, 1 out]
            }
            frame False {
              n147 = To Variant(anything=variant ("variant")) -> (Variant=w619:variant)
            }
          }
        }
      }
    }
    frame True {
      # "String or Path"
      n148 = String Length(string=w620) -> (length=w627:i32)
      n149 = Decrement(x=w627) -> (x-1=w623:i32)
      n150 = String Subset(string=w620, offset (0)=w623, length (rest)=1 ("length (rest)")) -> (substring=w624:string)
      n151 = Equal?(x=w624, y="\"" ("x")) -> (x = y?=w622:bool)
      n152 = case shown="True" w622 {
        tunnel: [_ w631] -> w628
        tunnel: w620 -> [_ w642]
        tunnel: w623 -> [_ w641]
        tunnel: [Character_Class_--_Enum."Invalid" w630] -> w621
        frame False {
        }
        frame True {
          n153 = Decrement(x=w641) -> (x-1=w640:i32)
          n154 = String Subset(string=w642, offset (0)=1, length (rest)=w640) -> (substring=w632:string)
          n155 = String Subset(string=w632, length (rest)=1 ("length (rest)")) -> (substring=w638:string)  [unwired: 1 in]
          n156 = Equal?(x="/", y=w638) -> (x = y?=w636:bool)
          n157 = Select(t=u8 50 ("Type"), s=w636, f=u8 48 ("Type")) -> (s? t:f=w633:u8)
          n158 = case shown="32" w633 {
            tunnel: [w647 w650] -> w631
            tunnel: w632 -> [w646 w648]
            tunnel: [Character_Class_--_Enum."Path" Character_Class_--_Enum."String"] -> w630
            frame 50 {
              # "PATH (0x32)"
              n159 = call "Common Path to Specific Path.vi"("common path"=w646) -> ("specific path"=w645:path)  [unwired: 10 in]
              n160 = To Variant(anything=w645) -> (Variant=w647:variant)
            }
            frame 48, Default {
              # "STRING (0x30)"
              n161 = To Variant(anything=w648) -> (Variant=w650:variant)
            }
          }
        }
      }
    }
  }
  "Variant-formatted Value" <- w9
  "Value Class" <- w3
